vi "TwoWheelObject.vi"(11 "Robot Configuration":T1={"wheel parameters"={"wheel radius"=0.05, "gear ratio"=1.0, "forward rotation direction"=0}, "wheel separation"=0.4, "Encoder Pulse Per Rev"=1856.0, "Update Period (sec)"=20.0, "Initial posture frame"=[0.0, 0.0, 0.0]} {"wheel parameters"."forward rotation direction" items=["Clockwise", "Counterclockwise"]}) -> (0 "error out":errorcluster, 3 "differential steering frame out":refnum<class "NI_Robotics_Differential Steering Frame.lvclass">)   [LabVIEW 2016]
uses:
  <vilib>/robotics/Steering/Differential Steering Frame/NI_Robotics_Differential Steering Frame.lvclass
  MotorControl/Configurations.ctl
  <vilib>/robotics/Steering/Wheel/Wheel Parameters.ctl
  <vilib>/robotics/Steering/Wheel/Rotation Direction.ctl
  <vilib>/robotics/Steering/Fixed Wheel/Create Fixed Wheel.vi
  <vilib>/robotics/Steering/Differential Steering Frame/Create Differential Steering Frame.vi
  <vilib>/robotics/Steering/Steering Frame/NI_Robotics_Steering Frame.lvclass
  <vilib>/robotics/Steering/Wheel/NI_Robotics_Wheel.lvclass
  <vilib>/robotics/Steering/Fixed Wheel/NI_Robotics_Fixed Wheel.lvclass
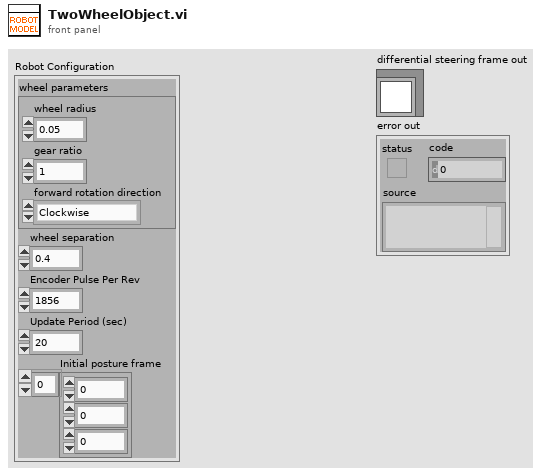
[diagram p1: front panel]
types:
  T1 = typedef "Configurations.ctl" = cluster{"wheel parameters":T2, "wheel separation":dbl, "Encoder Pulse Per Rev":dbl, "Update Period (sec)":dbl, "Initial posture frame":dbl[]}
  T2 = typedef "NI_Robotics_Wheel.lvclass/Wheel Parameters.ctl" = cluster{"wheel radius":dbl, "gear ratio":dbl, "forward rotation direction":T3}
  T3 = typedef "NI_Robotics_Wheel.lvclass/Rotation Direction.ctl" = u16
  T4 = cluster{"fixed wheel out":refnum<class "NI_Robotics_Fixed Wheel.lvclass">, "fixed wheel out":refnum<class "NI_Robotics_Fixed Wheel.lvclass">}
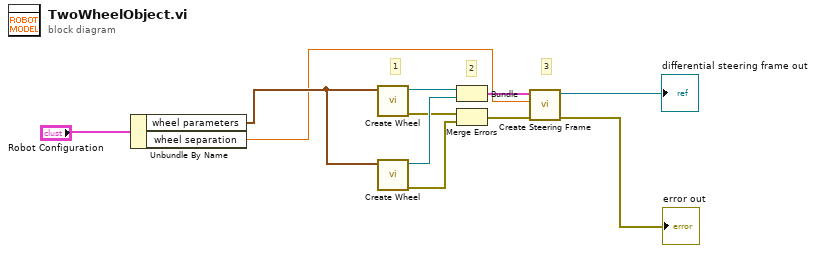
[diagram p0: block diagram]
diagram:
  # "3"
  # "2"
  # "1"
  n1 = Unbundle By Name("Robot Configuration") -> ("wheel parameters"=w3:T2, "wheel separation"=w2:dbl)
  n2 = call-poly <vilib>:"Create Wheel.vi"("wheel parameters"=w3) -> ("error out"=w8:errorcluster, "fixed wheel out"=w11:refnum<class "NI_Robotics_Fixed Wheel.lvclass">)  [unwired: 9 in]
  n3 = call-poly <vilib>:"Create Wheel.vi"("wheel parameters"=w3) -> ("error out"=w7:errorcluster, "fixed wheel out"=w10:refnum<class "NI_Robotics_Fixed Wheel.lvclass">)  [unwired: 9 in]
  n4 = Bundle("fixed wheel out"=w11, "fixed wheel out"=w10) -> (w9:T4)  [unwired: 1 in]
  n5 = Merge Errors(w8, w7) -> (w6:errorcluster)
  n6 = call-poly <vilib>:"Create Steering Frame.vi"("error in (no error)"=w6, "wheel separation"=w2, "wheels"=w9) -> ("error out"=→"error out":errorcluster, "differential steering frame out"=→"differential steering frame out":refnum<class "NI_Robotics_Differential Steering Frame.lvclass">)  [unwired: 7 in]
